vi "Furnace PID SP 1.vi"(6 "PID gains":T1={"proportional gain (Kc)"=1.0, "integral time (Ti, min)"=0.1, "derivative time (Td, min)"=0.0}, 8 "PV deg C":dbl format="%.2f", 9 "User SP Deg C":dbl format="%.2f") -> (2 "output T SP":dbl format="%.2f", 5 "Test Probe":dbl[](array[numeric]))   [LabVIEW 2014]
uses:
  <vilib>/addons/control/pid/pid.llb/PID (DBL).vi
  <vilib>/addons/control/pid/NI_PID_pid.lvlib
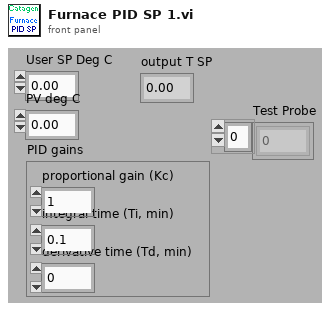
[diagram p1: front panel]
types:
  T1 = cluster{"proportional gain (Kc)":dbl, "integral time (Ti, min)":dbl, "derivative time (Td, min)":dbl}
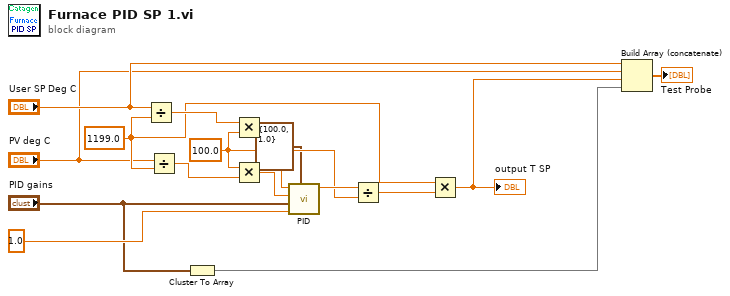
[diagram p0: block diagram]
diagram:
  w10 = 100.0 ("upper limit")
  w8 = 1199.0 ("upper limit")
  n1 = Divide(x="User SP Deg C", y=w8) -> (x/y=w12:dbl)
  n2 = Divide(x="PV deg C", y=w8) -> (x/y=w14:dbl)
  n3 = Cluster To Array(cluster="PID gains") -> (array=w3:dbl[])
  n4 = Multiply(x=w12, y=w10) -> (x*y=w13:dbl)
  n5 = Multiply(x=w10, y=w14) -> (x*y=w15:dbl)
  n6 = call-poly <vilib>:"PID.vi"("output range"=cluster{"output high":dbl, "output low":dbl} {"output high"=100.0, "output low"=1.0}, "dt (s)"=1.0, "PID gains"="PID gains", "process variable"=w15, "setpoint"=w13) -> ("output"=w11:dbl)  [unwired: 5 in, 1 out]
  n7 = Divide(x=w11, y=w10) -> (x/y=w9:dbl)
  n8 = Multiply(x=w8, y=w9) -> (x*y=w5:dbl)
  "output T SP" <- w5
  n9 = Build Array (concatenate)("User SP Deg C", "PV deg C", w5, w3) -> (→"Test Probe":dbl[])
